vi "MoveRef.vi"(8 "error in":errorcluster, 9 "Axis":i32, 10 "Position":dbl, 11 "VISA resource":refnum<visa-resource-name>) -> (0 "error out":errorcluster)   [LabVIEW 2012, in "Micos_uic.lvlib"]
uses:
  <instrlib>/Micos_uic/Micos_uic.lvlib
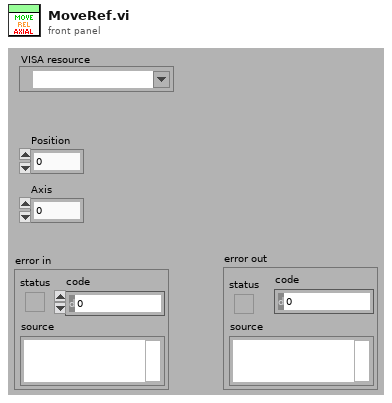
[diagram p1: front panel]
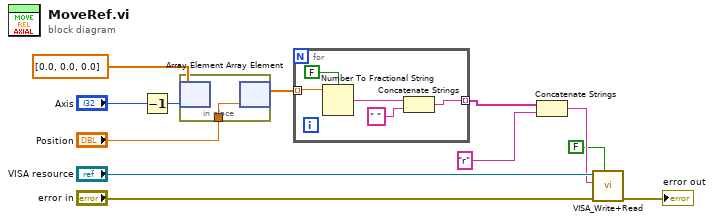
[diagram p0: block diagram]
diagram:
  n1 = Decrement(x="Axis") -> (x-1=w9:i32)
  n2 = in-place {
    in-place-border: "Position" -> [w13]
    n3 = in-place-array #1(dbl[] [0.0, 0.0, 0.0] ("Position_Micos"), w9) -> ()  [unwired: 1 out]
    n4 = in-place-array #1(w13) -> (w8:dbl[])  [unwired: 1 out]
  }
  n5 = for {
    tunnel: w8 -> [w18] mode=indexing
    tunnel: [w14] -> w6 mode=indexing
    n6 = Number To Fractional String(use system decimal point (T)=FALSE, number=w18) -> (F-format string=w16:string)  [unwired: 2 in]
    n7 = Concatenate Strings(w16, " " ("string")) -> (w14:string)
  }
  n8 = Concatenate Strings(w6, "r" ("format string")) -> (w3:string)
  n9 = call <instrlib>:"VISA_Write+Read.vi"("Read?"=FALSE, "error in (no error)"="error in", "Write Buffer"=w3, "VISA resource name"="VISA resource") -> ("error out"=→"error out":errorcluster)  [unwired: 5 in, 2 out]
